vi "Read Config.vi"(8 "error in (no error)":errorcluster, 10 "Resource In":variant, 11 "Width Method in":refnum<class "Width Method.lvclass">) -> (0 "error out":errorcluster, 2 "Resource Out":variant, 3 "Width Method out":refnum<class "Width Method.lvclass">)   [LabVIEW 2014, in "Width Method.lvclass"]
uses:
  Width Method.lvclass
  Utility/Width Method.ctl
  <vilib>/Utility/config.llb/Config Data RefNum.ctl
  Width Method.lvclass/Width Method.ctl
  <vilib>/Utility/config.llb/Read Key (String).vi
  <vilib>/Utility/config.llb/NI_LVConfig.lvlib
  Utility/POLARIS Vision utility.lvlib
panel:
  in  "Method":T1
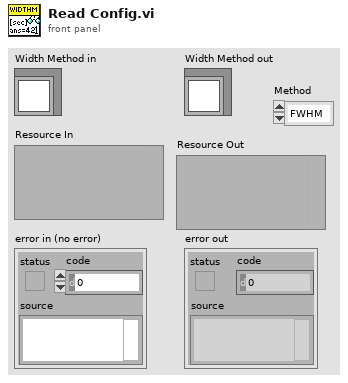
[diagram p1: front panel]
types:
  T1 = typedef "POLARIS Vision utility.lvlib/Width Method.ctl" = enum16{"FWHM", "1/e", "1/e^2", "80%", "90%"}
  T2 = typedef "NI_LVConfig.lvlib/Config Data RefNum.ctl" = refnum<k1>
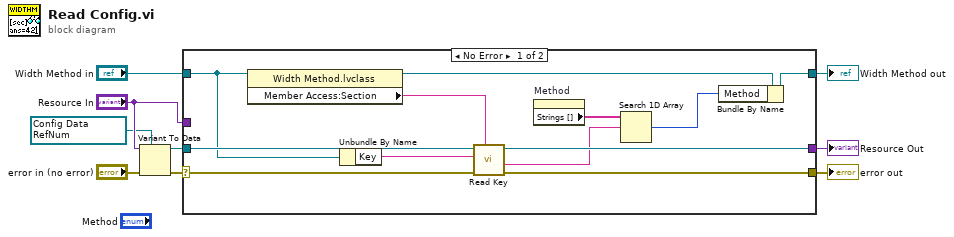
[diagram p0: block diagram]
diagram:
  w6 = T2 refnum items=["config data"] ("refnum")
  n1 = Variant To Data(error in="error in (no error)", type=w6, Variant="Resource In") -> (data=w5:T2, error out=w8:errorcluster)
  n2 = case shown="No Error" w8 {
    selector: w8 -> [w14 w23]
    tunnel: w5 -> [w21 _]
    tunnel: "Width Method in" -> [w15 w22]
    tunnel: [w18 w22] -> w3
    tunnel: [w19 w24] -> w2
    tunnel: [w13 w23] -> w1
    tunnel: "Resource In" -> [_ w24]
    frame No Error {
      n3 = property class="Width Method.lvclass"(reference=w15) -> (reference out=w16:refnum<class "Width Method.lvclass">, "Member Access:Section"=w20:string)  [unwired: 1 in, 1 out]
      n4 = Unbundle By Name(w15) -> ("Key"=w17:string)
      n5 = call-poly <vilib>:"Read Key.vi"("section"=w20, "error in (no error)"=w14, "key"=w17, "refnum"=w21) -> ("error out"=w13:errorcluster, "value"=w11:string, "refnum out"=w19:T2)  [unwired: 4 in, 1 out]
      n6 = property on="Method" class="Enum (strict)"() -> ("Strings []"=w12:string[])  [unwired: 2 in, 2 out]
      n7 = Search 1D Array(1D array=w12, element=w11) -> (index of element=w10:i32)  [unwired: 1 in]
      n8 = Bundle By Name(cluster=w16, "Method"=w10) -> (w18:refnum<class "Width Method.lvclass">)
    }
    frame Error {
    }
  }
  "error out" <- w1
  "Width Method out" <- w3
  "Resource Out" <- w2
